vi "Actor Core.vi"(8 "error in":errorcluster, 11 "client in":refnum<class "client.lvclass">) -> (0 "error out":errorcluster, 3 "Actor out":refnum<class "Actor.lvclass">)   [LabVIEW 2016, in "client.lvlib" / "client.lvclass"]
doc: "(<B>Filename</B>: Actor Framework.lvlib:Actor.lvclass:Actor Core.vi)\n\nReceives messages to the actor, reacts to them, and initiates any error handling that may shut the actor down.\n\nDescendant classes may override this VI to append parallel tasks for the actor to complete while it handles messages. Overrides use the Call Parent Method node."
uses:
  client.lvclass
  C:/Program Files/National Instruments/LabVIEW 2016/vi.lib/ActorFramework/Actor/Actor.lvclass
  <vilib>/ActorFramework/Actor/Actor.lvclass
  <vilib>/ActorFramework/Actor/Actor.lvclass/Actor.ctl
  <vilib>/ActorFramework/Message Enqueuer/Message Enqueuer.lvclass/Message Enqueuer.ctl
  client.lvclass/client.ctl
  server/server Messages/send message to server Msg/send message to server Msg.lvclass/send message to server Msg.ctl
  <vilib>/ActorFramework/Message Enqueuer/Init from Existing Queue.vi
  <vilib>/ActorFramework/Message Enqueuer/Enqueue.vi
  <vilib>/ActorFramework/Stop Msg/Stop Msg.lvclass
  C:/Program Files/National Instruments/LabVIEW 2016/vi.lib/ActorFramework/Message/Message.lvclass
  server/server Messages/send message to server Msg/send message to server Msg.lvclass
  <vilib>/ActorFramework/Message Priority Queue/Priority Enqueue.vi
  <vilib>/ActorFramework/Message Enqueuer/Message Enqueuer.lvclass
panel:
  out "ID":string
  in  "send":bool=TRUE
  in  "msg to send":string
  in  "stop":bool=TRUE
  # "Client"
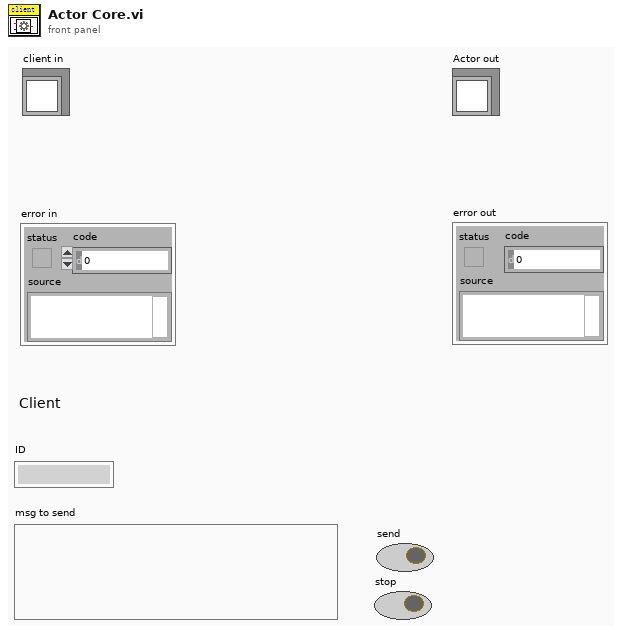
[diagram p1: front panel]
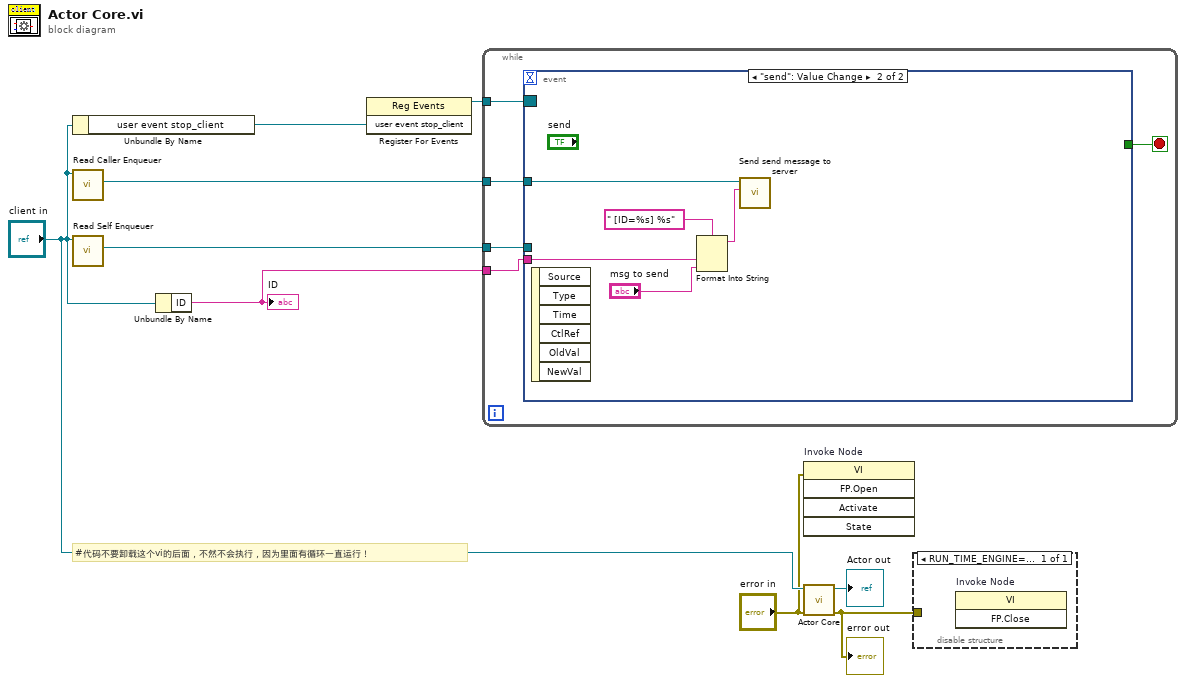
[diagram p0: block diagram]
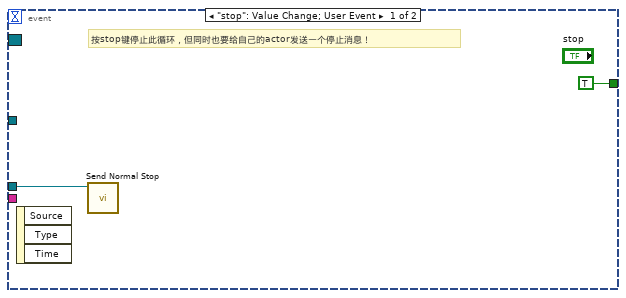
[diagram p2: hidden frame]
diagram:
  # "#代码不要卸载这个vi的后面，不然不会执行，因为里面有循环一直运行！"
  n1 = Unbundle By Name("client in") -> ("user event stop_client"=w3:refnum<user-event>)
  n2 = call <vilib>:"Read Caller Enqueuer.vi"("Actor"="client in") -> ("Caller Enqueuer"=w6:refnum<class "Message Enqueuer.lvclass">)  [unwired: 10 in]
  n3 = call <vilib>:"Read Self Enqueuer.vi"("Actor"="client in") -> ("Self Enqueuer"=w7:refnum<class "Message Enqueuer.lvclass">)  [unwired: 10 in]
  n4 = Unbundle By Name("client in") -> ("ID"=w4:string)
  "ID" <- w4
  n5 = register-events(w3) -> (reference out=w8:refnum<event-registration>)  [unwired: 2 in, 1 out]
  n6 = while {
    tunnel: w8 -> [w13]
    tunnel: w7 -> [w12]
    tunnel: w6 -> [w11]
    tunnel: w4 -> [w10]
    stop <- w14 stop-if-true
    n7 = event shown="[1] \"send\": Value Change" {
      selector: w13 -> [_ _]
      dyn-events: _ -> [_ _]
      timeout: _ -> [_ _]
      tunnel: [TRUE _] -> w14
      tunnel: w12 -> [w15 _]
      tunnel: w11 -> [_ w21]
      tunnel: w10 -> [_ w18]
      event "stop": Value Change; User Event {
        # "按stop键停止此循环，但同时也要给自己的actor发送一个停止消息！"
        n8 = event-data() -> ()  [unwired: 1 in, 3 out]
        n9 = call <vilib>:"Send Normal Stop.vi"("Message Enqueuer"=w15) -> ()  [unwired: 10 in, 1 out]
      }
      event "send": Value Change {
        n10 = event-data() -> ()  [unwired: 1 in, 6 out]
        n11 = Format Into String(format string=" [ID=%s] %s", w18, "msg to send") -> (resulting string=w19:string)  [unwired: 2 in, 1 out]
        n12 = call "Send send message to server.vi"("event message"=w19, "Message Enqueuer"=w21) -> ()  [unwired: 8 in, 2 out]
      }
    }
  }
  n13 = invoke on="Invoke Node" class="VI" method="FP.Open"(error in="error in") -> ()  [unwired: 4 in, 5 out]
  n14 = call-parent "Actor Core.vi"("error in"="error in", "Actor in"="client in") -> ("error out"=w2:errorcluster, "Actor out"=→"Actor out":refnum<class "Actor.lvclass">)  [unwired: 8 in]
  "error out" <- w2
  n15 = disable-structure shown="RUN_TIME_ENGINE==True, Default" {
    disable-tunnel: w2 -> [_]
    frame condition #0 (active) {
      n16 = invoke on="Invoke Node" class="VI" method="FP.Close"() -> ()  [unwired: 3 in, 3 out]
    }
  }
